vi "[GV]_IMU acceleration.vi"() -> ()   [LabVIEW 2016]
panel:
  in  "IMU Acceleration":dbl
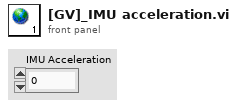
[diagram p1: front panel]
diagram:
